vi "rad_RunImageConversion.vi"(4 "error in":errorcluster, 7 "Image Path":path) -> (0 "error out":errorcluster)   [LabVIEW 2020]
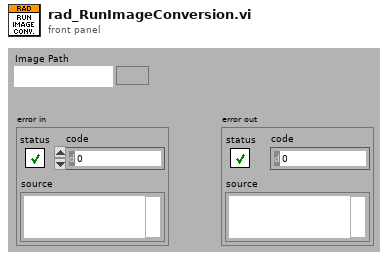
[diagram p1: front panel]
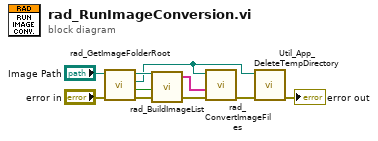
[diagram p0: block diagram]
diagram:
  n1 = call "rad_GetImageFolderRoot.vi"("error in"="error in", "Image Path"="Image Path") -> ("error out"=w1:errorcluster, "directory"=w4:bool, "ImageFolderRoot"=w2:path, "Image Path out"=w8:path)  [unwired: 2 in]
  n2 = call "rad_BuildImageList.vi"("error in"=w1, "directory"=w4, "Image Path"=w8) -> ("error out"=w5:errorcluster, "filenames"=w3:string[])  [unwired: 1 in]
  n3 = call "rad_ConvertImageFiles.vi"("error in"=w5, "ImageFiles"=w3, "ImageFolderRoot"=w2) -> ("error out"=w9:errorcluster)  [unwired: 4 in]
  n4 = call "Util_App_DeleteTempDirectory.vi"("error in"=w9, "RootFolder"=w2) -> ("error out"=→"error out":errorcluster)  [unwired: 5 in]
